vi "oa_Process Order Power Spectrum (1 Channel).vi"(0 "resampled signal":cluster{"r0":dbl, "dr":dbl, "Y":dbl[]}={"r0"=0.0, "dr"=1.0, "Y"=[]} {"r0" format="%.2p"; "dr" format="%.2p"; "Y" format="%.2f"}, 5 "resampled channel info":T9={"channel name"="", "description"="", " channel info"={"sensor sensitivity"=1000.0, "engineering units"=1, "dB reference"=1.0, "custom label"="EU", "weighting filter"=0, "pregain"=0.0}} {"channel info"."pregain" format="%.2f"; "channel info"."weighting filter" items=["Linear", "A-weighting", "B-weighting", "C-weighting", "ITU-R 468-4", "Dolby", "CCITT", "C-message", "Wb", "Wc", "Wd", "We", "Wf", "Wh", "Wj", "Wk", "Wm", "AES17 20 kHz lowpass", "AES17 40 kHz lowpass", "AES17 20 kHz highpass", "AES17 40 kHz highpass"]; "channel info"."dB reference" format="%^.1e"; "channel info"."engineering units" items=["custom..."=0, "V"=1, "A"=21, "C"=30, "pC"=31, "s"=32, "-"=29, "Pa"=2, "N"=20, "g"=3, "m/s^2"=4, "m/s"=5, "m"=6, "mm/s"=12, "mm"=13, "micron/s"=14, "micron"=15, "in/s^2"=7, "in/s"=8, "in"=9, "mil/s"=10, "mil"=11, "rad/s^2"=16, "rad/s"=17, "rad"=18, "deg/s^2"=26, "deg/s"=27, "deg"=28, "RPM"=22, "cycle/s^2"=23, "Hz"=24, "cycle"=25, "strain"=19]; "channel info"."sensor sensitivity" format="%#_5f"}, 7 "spectrum settings":cluster{"window type":u32, "block size":i32}={"window type"=1, "block size"=200} {"block size" min=2; "window type" items=["None"=0, "Hanning"=1, "Hamming"=2, "Blackman-Harris"=3, "Exact Blackman"=4, "Blackman"=5, "Flat Top"=6, "4 Term B-Harris"=7, "7 Term B-Harris"=8, "Low Sidelobe"=9, "Gaussian"=62]}, 9 "averaging parameters":T11={"averaging mode"=enum."No averaging", "weighting mode"=enum."Exponential", "number of averages"=10, "linear mode"=enum."One shot"} {"number of averages" min=1 step=1}, 11 "error in":errorcluster, 12 "processing control in":T1(ring)) -> (2 "new spectrum available?":bool, 3 "averages completed":dbl, 4 "order spectrum":T8={"order 0"=0.0, "delta order"=1.0, "magnitude"=[]} {"order 0" format="%.2p"; "delta order" format="%.2p"; "magnitude" format="%.2f"}, 8 "averaging done":bool, 10 "spectrum info":T2={"channel name"="", "description"="", "x-axis units"=0, "spectral info"={"spectrum type"=enum."Power [Magnitude^2]", "linear/dB"=enum."linear", "window"=0, "window size"=0, "FFT size"=0}, "engineering units"=1, "custom label"="", "dB reference [EU]"=0.0, "peak units"=enum."rms", "weighting filter"=0, "spectral density?"=FALSE, "unit label"="", "spectrum skewed?"=FALSE, "complimentary spectrum units"=enum."none"} {"x-axis units" items=["Time (s)"=0, "Frequency-CB (Hz)"=1, "Frequency-CPB (Hz)"=1248, "Frequency-Arbitrary (Hz)"=2357, "Quefrency (s)"=2, "Revolutions (rev)"=3, "Order"=4, "Speed (RPM)"=11, "Speed (rad/s)"=21, "Index"=65535]; "weighting filter" items=["Linear", "A-weighting", "B-weighting", "C-weighting", "ITU-R 468-4", "Dolby", "CCITT", "C-message", "Wb", "Wc", "Wd", "We", "Wf", "Wh", "Wj", "Wk", "Wm", "AES17 20 kHz lowpass", "AES17 40 kHz lowpass", "AES17 20 kHz highpass", "AES17 40 kHz highpass"]; "dB reference [EU]" format="%.2f"; "engineering units" items=["custom..."=0, "V"=1, "A"=21, "C"=30, "pC"=31, "s"=32, "-"=29, "Pa"=2, "N"=20, "g"=3, "m/s^2"=4, "m/s"=5, "m"=6, "mm/s"=12, "mm"=13, "micron/s"=14, "micron"=15, "in/s^2"=7, "in/s"=8, "in"=9, "mil/s"=10, "mil"=11, "rad/s^2"=16, "rad/s"=17, "rad"=18, "deg/s^2"=26, "deg/s"=27, "deg"=28, "RPM"=22, "cycle/s^2"=23, "Hz"=24, "cycle"=25, "strain"=19]; "spectral info"."window" items=["None "=0, "Hanning"=1, "Hamming"=2, "Blackman-Harris"=3, "Exact Blackman"=4, "Blackman"=5, "Flat Top"=6, "4 Term B-Harris "=7, "7 Term B-Harris"=8, "Low Sidelobe"=9, "Force - Exponential"=10, "Gaussian"=62]}, 14 "processing control out":T1(ring), 15 "error out":errorcluster)   [LabVIEW 2017, in "SoundVib_Resampling.lvlib"]
uses:
  <vilib>/addons/Sound and Vibration/Order Analysis/Resample Order Tracking/SoundVib_Resampling.lvlib
  <vilib>/addons/_NISVFA/_Shared subVIs/Controls/svc_Resampled Channel Info.ctl
  <vilib>/addons/_NISVFA/_Shared subVIs/Controls/svc_Channel Info.ctl
  <vilib>/addons/_NISVFA/_Shared subVIs/Controls/svc_Engineering Units Text Ring.ctl
  <vilib>/addons/_NISVFA/_Shared subVIs/Controls/svc_Weighting Filter Text Ring.ctl
  <vilib>/addons/_NISVFA/_Shared subVIs/Controls/svc_Spectrum Info.ctl
  <vilib>/addons/_NISVFA/_Shared subVIs/Controls/svc_X-Axis Units.ctl
  <vilib>/addons/_NISVFA/_Shared subVIs/Controls/svc_Spectrum Type.ctl
  <vilib>/addons/_NISVFA/_Shared subVIs/Controls/svc_Complimentary Spectrum Units.ctl
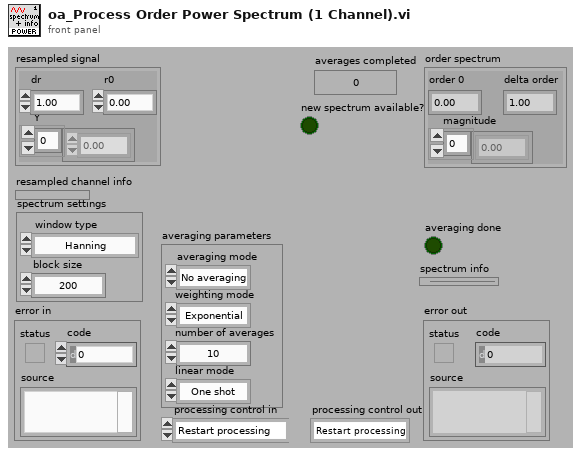
[diagram p1: front panel]
types:
  T1 = enum16{"Restart processing", "Continue processing", "Skip processing"}
  T2 = typedef "svc_Spectrum Info.ctl" = cluster{"channel name":string, "description":string, "x-axis units":T3, "spectral info":cluster{"spectrum type":T4, "linear/dB":enum16{"linear", "dB"}, "window":u16, "window size":i32, "FFT size":i32}, "engineering units":T5, "custom label":string, "dB reference [EU]":dbl, "peak units":enum16{"rms", "peak", "peak-peak"}, "weighting filter":T6, "spectral density?":bool, "unit label":string, "spectrum skewed?":bool, "complimentary spectrum units":T7}
  T3 = typedef "svc_X-Axis Units.ctl" = u16
  T4 = typedef "svc_Spectrum Type.ctl" = enum16{"FFT Spectrum [complex]", "Amplitude [Magnitude]", "Power [Magnitude^2]", "Cross Spectrum [complex]", "Frequency Response [Complex]"}
  T5 = typedef "svc_Engineering Units Text Ring.ctl" = u16
  T6 = typedef "svc_Weighting Filter Text Ring.ctl" = u16
  T7 = typedef "svc_Complimentary Spectrum Units.ctl" = enum16{"none", "radians", "degrees", "cycles", "imaginary"}
  T8 = cluster{"order 0":dbl, "delta order":dbl, "magnitude":dbl[]}
  T9 = typedef "svc_Resampled Channel Info.ctl" = cluster{"channel name":string, "description":string, " channel info":T10}
  T10 = typedef "svc_Channel Info.ctl" = cluster{"sensor sensitivity":dbl, "engineering units":T5, "dB reference":dbl, "custom label":string, "weighting filter":T6, "pregain":dbl}
  T11 = cluster{"averaging mode":enum16{"No averaging", "Vector averaging", "RMS averaging", "Peak hold"}, "weighting mode":enum16{"Linear", "Exponential"}, "number of averages":u32, "linear mode":enum16{"One shot", "Auto restart"}}
  T12 = cluster{"complex FFT":cdb[], "power spectrum":dbl[], "averages completed":dbl}
  T13 = enum16{"No averaging", "Vector averaging", "RMS averaging", "Peak hold"}
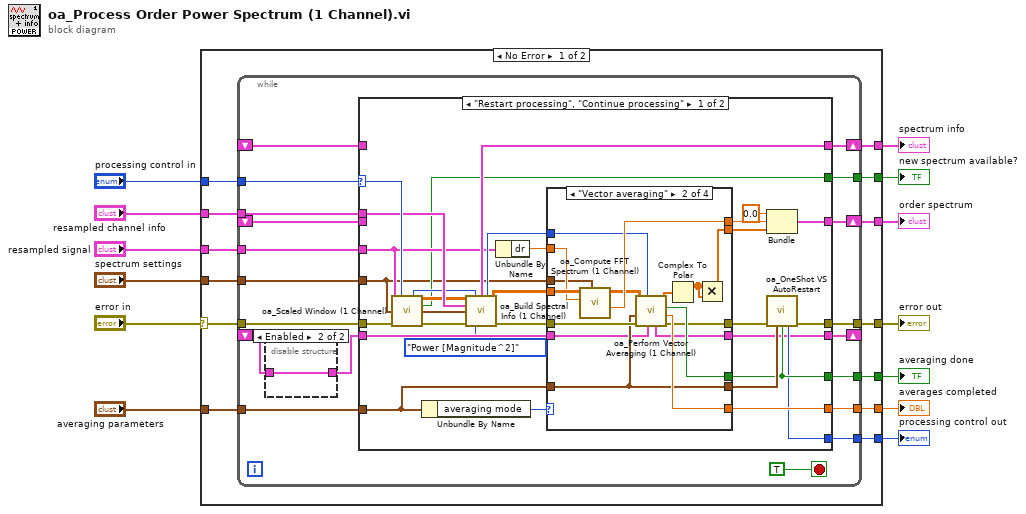
[diagram p0: block diagram]
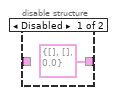
[diagram p2: hidden frame]
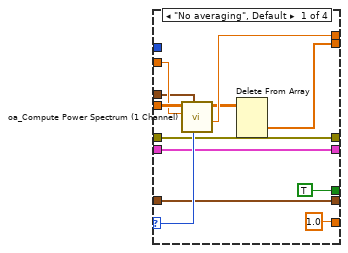
[diagram p3: hidden frame]
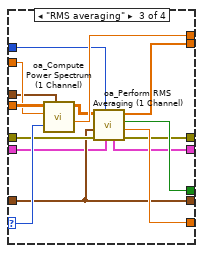
[diagram p4: hidden frame]
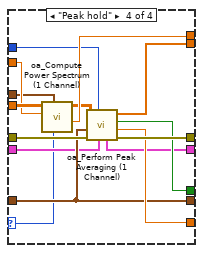
[diagram p5: hidden frame]
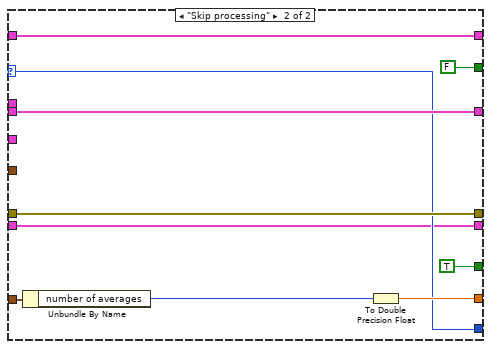
[diagram p6: hidden frame]
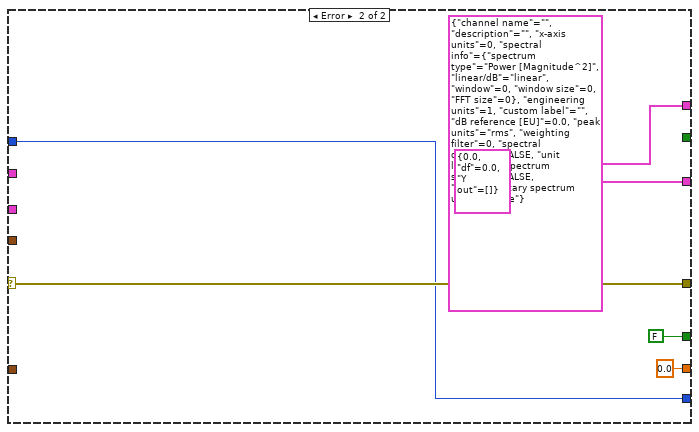
[diagram p7: hidden frame]
diagram:
  n1 = case shown="No Error" "error in" {
    selector: "error in" -> [w25 w151]
    tunnel: [w19 w151] -> w12
    tunnel: "resampled signal" -> [w26 _]
    tunnel: "spectrum settings" -> [w24 _]
    tunnel: "processing control in" -> [w23 w146]
    tunnel: "resampled channel info" -> [w22 _]
    tunnel: "averaging parameters" -> [w21 _]
    tunnel: [w20 T2 {"channel name"="", "description"="", "x-axis units"=0, "spectral info"={"spectrum type"=enum."Power [Magnitude^2]", "linear/dB"=enum."linear", "window"=0, "window size"=0, "FFT size"=0}, "engineering units"=1, "custom label"="", "dB reference [EU]"=0.0, "peak units"=enum."rms", "weighting filter"=0, "spectral density?"=FALSE, "unit label"="", "spectrum skewed?"=FALSE, "complimentary spectrum units"=enum."none"} ("spectrum info")] -> w6
    tunnel: [w18 0.0 ("averages completed")] -> w5
    tunnel: [w17 FALSE ("averaging done")] -> w4
    tunnel: [w16 cluster{dbl, "df":dbl, "Y out":dbl[]} {0.0, "df"=0.0, "Y out"=[]}] -> w3
    tunnel: [w15 w146] -> w2
    tunnel: [w14 _] -> w1
    frame No Error {
      n2 = while {
        tunnel: w26 -> [w44]
        tunnel: w25 -> [w43]
        tunnel: w24 -> [w42]
        tunnel: w23 -> [w41]
        tunnel: w22 -> [w40]
        tunnel: w21 -> [w39]
        shift-right: [w38] -> w20
        shift-left: _ -> [w37]
        tunnel: [w36] -> w19
        tunnel: [w35] -> w18
        tunnel: [w34] -> w17
        shift-right: [w33] -> w16
        shift-left: _ -> [w32]
        tunnel: [w31] -> w15
        shift-right: [w30] -> _
        shift-left: _ -> [w27]
        tunnel: [w29] -> w14
        stop <- TRUE stop-if-true
        n3 = disable-structure shown="Enabled" {
          disable-tunnel: [T12 {"complex FFT"=[], "power spectrum"=[], "averages completed"=0.0} ("averaging state info out") w47] -> w28
          disable-tunnel: w27 -> [_ w47]
          frame Disabled {
          }
          frame Enabled {
          }
        }
        n4 = case shown="\"Restart processing\", \"Continue processing\"" w41 {
          selector: w41 -> [w76 w138]
          tunnel: w44 -> [w65 _]
          tunnel: w43 -> [w77 w144]
          tunnel: w42 -> [w48 _]
          tunnel: w40 -> [w73 _]
          tunnel: w39 -> [w51 w142]
          tunnel: [w67 w145] -> w38
          tunnel: w37 -> [_ w145]
          tunnel: [w58 w144] -> w36
          tunnel: [w63 w140] -> w35
          tunnel: [w56 TRUE ("averaging done")] -> w34
          tunnel: [w50 w139] -> w33
          tunnel: w32 -> [_ w139]
          tunnel: [w55 w138] -> w31
          tunnel: [w54 w137] -> w30
          tunnel: w28 -> [w53 w137]
          tunnel: [w49 FALSE ("new spectrum available?")] -> w29
          frame "Restart processing", "Continue processing" {
            n5 = call <vilib>:"oa_Scaled Window (1 Channel).vi"("resampled signal"=w65, "processing control in"=w76, "spectrum settings"=w48, "error in"=w77) -> ("dup processing control"=w72:T1, "Y"=w70:dbl[][], "new spectrum available?"=w49:bool, "spectrum settings"=w74:cluster{"window type":u32, "block size":i32}, "error out"=w75:errorcluster)  [unwired: 7 in]
            n6 = Unbundle By Name(w51) -> ("averaging mode"=w71:T13)
            n7 = call <vilib>:"oa_Build Spectral Info (1 Channel).vi"("spectra in"=w70, "processing control in"=w72, "resampled channel info"=w73, "spectrum settings"=w74, "error in"=w75, "spectrum type"=svc_Spectrum_Type."Power [Magnitude^2]") -> ("spectrum info"=w67:T2, "dup processing control"=w66:T1, "spectra out"=w69:dbl[][], "error out"=w68:errorcluster)  [unwired: 6 in]
            n8 = Unbundle By Name(w65) -> ("dr"=w64:dbl)
            n9 = case shown="\"Vector averaging\"" w71 {
              selector: w71 -> [w87 _ w118 w122]
              tunnel: w69 -> [w89 w105 w120 w135]
              tunnel: w68 -> [w86 w102 w116 w131]
              tunnel: w66 -> [_ w100 w114 w129]
              tunnel: w64 -> [w88 w104 w119 w134]
              tunnel: [w78 w90 w113 w128] -> w62
              tunnel: [w86 w97 w110 w132] -> w59
              tunnel: w51 -> [w82 w96 w109 w125]
              tunnel: [1.0 ("averages completed") w98 w111 w126] -> w63
              tunnel: [TRUE ("averaging done") w99 w112 w127] -> w56
              tunnel: [w85 w103 w117 w133] -> w60
              tunnel: [w82 w96 w109 w125] -> w57
              tunnel: [w81 w94 w108 w124] -> w54
              tunnel: w53 -> [w81 w95 w107 w123]
              tunnel: w48 -> [w80 w93 w106 w121]
              frame "No averaging", Default {
                n10 = call <vilib>:"oa_Compute Power Spectrum (1 Channel).vi"("averaging mode"=w87, "spectrum settings"=w80, "dr"=w88, "Y"=w89) -> ("df"=w85:dbl, "power spectrum"=w79:dbl[][])  [unwired: 6 in]
                n11 = Delete From Array(array=w79) -> (deleted portion=w78:dbl[])  [unwired: 3 in, 1 out]
              }
              frame "Vector averaging" {
                n12 = call <vilib>:"oa_Compute FFT Spectrum (1 Channel).vi"("spectrum settings"=w93, "dr"=w104, "Y"=w105) -> ("df"=w103:dbl, "one-sided FFT spectrum"=w101:cdb[][])  [unwired: 7 in]
                n13 = call <vilib>:"oa_Perform Vector Averaging (1 Channel).vi"("averaging state info in"=w95, "processing control in"=w100, "error in (no error)"=w102, "averaging parameters"=w96, "Y"=w101) -> ("error out"=w97:errorcluster, "averages completed"=w98:dbl, "averaging done"=w99:bool, "Y out"=w91:cdb[], "averaging state info out"=w94:T12)  [unwired: 2 in]
                n14 = Complex To Polar(r * e^(i*theta)=w91) -> (r=w92:dbl[])  [unwired: 1 out]
                n15 = Multiply(x=w92, y=w92) -> (x*y=w90:dbl[])
              }
              frame "RMS averaging" {
                n16 = call <vilib>:"oa_Compute Power Spectrum (1 Channel).vi"("averaging mode"=w118, "spectrum settings"=w106, "dr"=w119, "Y"=w120) -> ("df"=w117:dbl, "power spectrum"=w115:dbl[][])  [unwired: 6 in]
                n17 = call <vilib>:"oa_Perform RMS Averaging (1 Channel).vi"("averaging state info in"=w107, "processing control in"=w114, "error in (no error)"=w116, "averaging parameters"=w109, "Y"=w115) -> ("error out"=w110:errorcluster, "averages completed"=w111:dbl, "averaging done"=w112:bool, "Y out"=w113:dbl[], "averaging state info out"=w108:T12)  [unwired: 2 in]
              }
              frame "Peak hold" {
                n18 = call <vilib>:"oa_Compute Power Spectrum (1 Channel).vi"("averaging mode"=w122, "spectrum settings"=w121, "dr"=w134, "Y"=w135) -> ("df"=w133:dbl, "power spectrum"=w130:dbl[][])  [unwired: 6 in]
                n19 = call <vilib>:"oa_Perform Peak Averaging (1 Channel).vi"("averaging state info out"=w123, "processing control in"=w129, "error in (no error)"=w131, "averaging parameters"=w125, "Y"=w130) -> ("error out"=w132:errorcluster, "averages completed"=w126:dbl, "averaging done"=w127:bool, "Y out"=w128:dbl[], "averaging state info out"=w124:T12)  [unwired: 2 in]
              }
            }
            n20 = Bundle(0.0, "df"=w60, "Y out"=w62) -> (w50:cluster{dbl, "df":dbl, "Y out":dbl[]})  [unwired: 1 in]
            n21 = call <vilib>:"oa_OneShot VS AutoRestart.vi"("error in (no error)"=w59, "averaging parameters"=w57, "averaging done"=w56) -> ("processing control out"=w55:T1, "error out"=w58:errorcluster)  [unwired: 11 in]
          }
          frame "Skip processing" {
            n22 = Unbundle By Name(w142) -> ("number of averages"=w141:u32)
            n23 = To Double Precision Float(number=w141) -> (double precision float=w140:dbl)
          }
        }
      }
    }
    frame Error {
    }
  }
  "order spectrum" <- w3
  "error out" <- w12
  "averaging done" <- w4
  "averages completed" <- w5
  "spectrum info" <- w6
  "processing control out" <- w2
  "new spectrum available?" <- w1
